vi "AddCommandFrame.vi"(5 "Command":T1 {"Data/Address/ByteCount" format="%.0x"}, 7 "Slave Address":u8 max=15 format="%.0x", 8 "error in (no error)":errorcluster, 9 "Number of Samples In":i32, 10 "Data Array In":u8[][](array[numeric]), 11 "RFFE_Data":T2 {"Toggle (high to low)" items=["0", "1", "Z", "L", "H", "X", "T", "V"]; "X Array" items=["0", "1", "Z", "L", "H", "X", "T", "V"]; "Z Array" items=["0", "1", "Z", "L", "H", "X", "T", "V"]; "L Array" items=["0", "1", "Z", "L", "H", "X", "T", "V"]; "H Array" items=["0", "1", "Z", "L", "H", "X", "T", "V"]; "One Array" items=["0", "1", "Z", "L", "H", "X", "T", "V"]; "Zero Array" items=["0", "1", "Z", "L", "H", "X", "T", "V"]}) -> (0 "error out":errorcluster, 1 "Number of Samples Out":i32, 2 "Data Array Out":u8[][](array[numeric]), 3 "Configuratation Out":T2 {"Toggle (high to low)" items=["0", "1", "Z", "L", "H", "X", "T", "V"]; "X Array" items=["0", "1", "Z", "L", "H", "X", "T", "V"]; "Z Array" items=["0", "1", "Z", "L", "H", "X", "T", "V"]; "L Array" items=["0", "1", "Z", "L", "H", "X", "T", "V"]; "H Array" items=["0", "1", "Z", "L", "H", "X", "T", "V"]; "One Array" items=["0", "1", "Z", "L", "H", "X", "T", "V"]; "Zero Array" items=["0", "1", "Z", "L", "H", "X", "T", "V"]})   [LabVIEW 2013]
doc: "Builds a MIPI RFFE command frame."
uses:
  Ctrls/RFFE_Data.ctl
  Ctrls/ClockDataChannels.ctl
  Ctrls/Commands.ctl
  Ctrls/Read_Write_Data.ctl
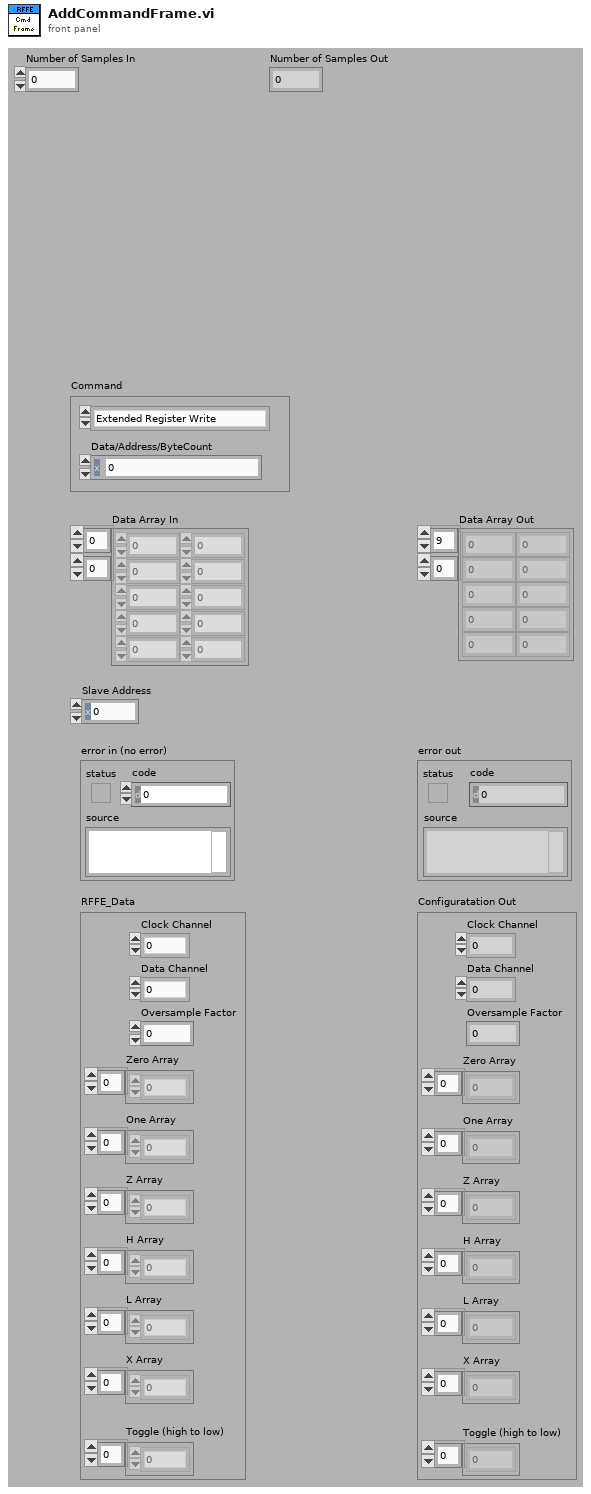
[diagram p1: front panel]
types:
  T1 = typedef "Commands.ctl" = cluster{"Command":enum16{"Extended Register Write", "Extended Register Read", "Extended Register Write Long", "Extended Register Read Long", "Register Write", "Register Read", "Register 0 Write"}, "Data/Address/ByteCount":u8}
  T2 = typedef "RFFE_Data.ctl" = cluster{"Clock Channel":T3, "Data Channel":T3, "Oversample Factor":u8, "Zero Array":u8[], "One Array":u8[], "Z Array ":u8[], "H Array":u8[], "L Array":u8[], "X Array":u8[], "Toggle (high to low)":u8[]}
  T3 = typedef "ClockDataChannels.ctl" = enum16{"0", "1"}
  T4 = enum16{"Extended Register Write", "Extended Register Read", "Extended Register Write Long", "Extended Register Read Long", "Register Write", "Register Read", "Register 0 Write"}
  T5 = typedef "Read_Write_Data.ctl" = cluster{"Data":u8, "Read/Write":enum16{"Read", "Write"}}
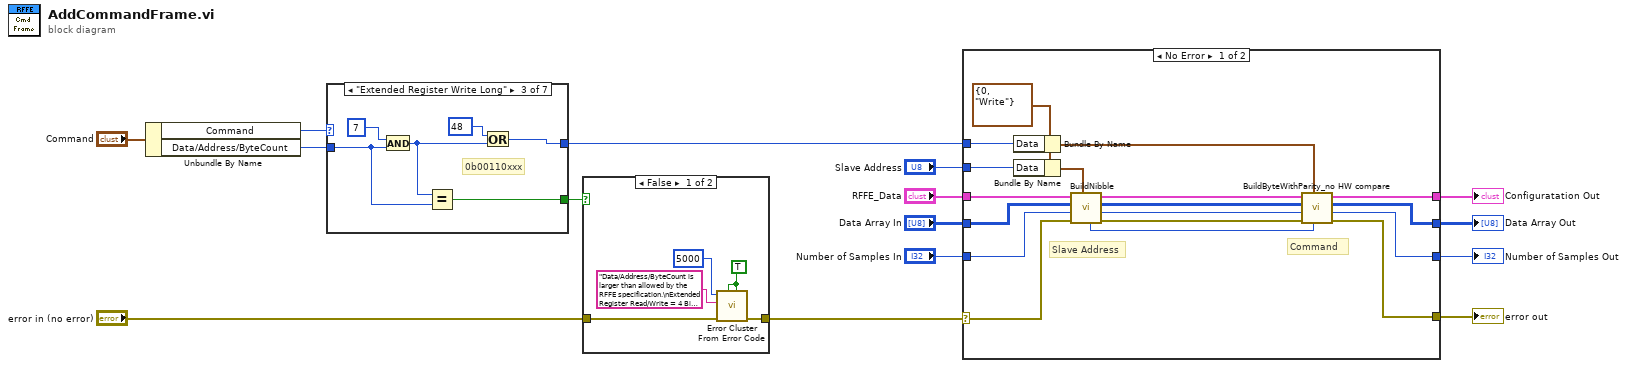
[diagram p0: block diagram]
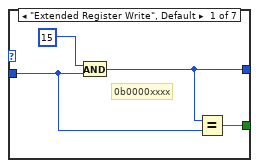
[diagram p3: hidden frame]
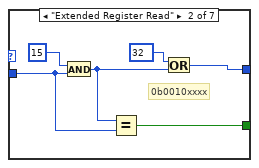
[diagram p4: hidden frame]
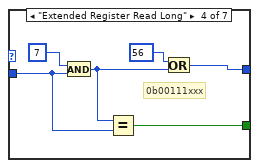
[diagram p5: hidden frame]
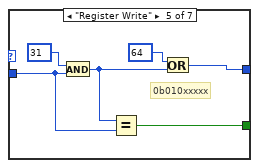
[diagram p6: hidden frame]
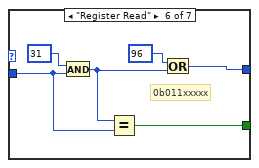
[diagram p7: hidden frame]
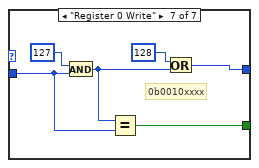
[diagram p8: hidden frame]
diagram:
  n1 = Unbundle By Name("Command") -> ("Command"=w9:T4, "Data/Address/ByteCount"=w8:u8)
  n2 = case shown="\"Extended Register Write Long\"" w9 {
    tunnel: w8 -> [w16 w20 w26 w32 w39 w45 w51]
    tunnel: [w17 w24 w29 w35 w41 w47 w53] -> w1
    tunnel: [w18 w22 w28 w34 w40 w44 w50] -> w7
    frame "Extended Register Write", Default {
      # "0b0000xxxx"
      n3 = And(x=u8 15, y=w16) -> (x .and. y?=w17:u8)
      n4 = Equal?(x=w17, y=w16) -> (x = y?=w18:bool)
    }
    frame "Extended Register Read" {
      # "0b0010xxxx"
      n5 = And(x=u8 15, y=w20) -> (x .and. y?=w21:u8)
      n6 = Equal?(x=w21, y=w20) -> (x = y?=w22:bool)
      n7 = Or(x=u8 32, y=w21) -> (x .or. y?=w24:u8)
    }
    frame "Extended Register Write Long" {
      # "0b00110xxx"
      n8 = And(x=u8 7, y=w26) -> (x .and. y?=w27:u8)
      n9 = Equal?(x=w27, y=w26) -> (x = y?=w28:bool)
      n10 = Or(x=u8 48, y=w27) -> (x .or. y?=w29:u8)
    }
    frame "Extended Register Read Long" {
      # "0b00111xxx"
      n11 = And(x=u8 7, y=w32) -> (x .and. y?=w33:u8)
      n12 = Equal?(x=w33, y=w32) -> (x = y?=w34:bool)
      n13 = Or(x=u8 56, y=w33) -> (x .or. y?=w35:u8)
    }
    frame "Register Write" {
      # "0b010xxxxx"
      n14 = And(x=u8 31, y=w39) -> (x .and. y?=w38:u8)
      n15 = Equal?(x=w38, y=w39) -> (x = y?=w40:bool)
      n16 = Or(x=u8 64, y=w38) -> (x .or. y?=w41:u8)
    }
    frame "Register Read" {
      # "0b011xxxxx"
      n17 = And(x=u8 31, y=w45) -> (x .and. y?=w46:u8)
      n18 = Equal?(x=w46, y=w45) -> (x = y?=w44:bool)
      n19 = Or(x=u8 96, y=w46) -> (x .or. y?=w47:u8)
    }
    frame "Register 0 Write" {
      # "0b0010xxxx"
      n20 = And(x=u8 127, y=w51) -> (x .and. y?=w52:u8)
      n21 = Equal?(x=w52, y=w51) -> (x = y?=w50:bool)
      n22 = Or(x=u8 128, y=w52) -> (x .or. y?=w53:u8)
    }
  }
  n23 = case shown="False" w7 {
    tunnel: [w59 w61] -> w5
    tunnel: "error in (no error)" -> [w60 w61]
    frame False {
      w56 = TRUE ("show call chain? (False)")
      n24 = call <vilib>:"Error Cluster From Error Code.vi"("is warning? (False)"=w56, "show call chain? (False)"=w56, "error in (no error)"=w60, "error message (\"\")"="Data/Address/ByteCount is larger than allowed by the RFFE specification.\nExtended Register Read/Write = 4 Bits\nExtended Register Read/Write Long = 3 Bits\nRegister Read/Write = 5 Bits\nRegister 0 Write = 7 Bits" ("error message (\"\")"), "error code (0)"=5000) -> ("error out"=w59:errorcluster)  [unwired: 4 in]
    }
    frame True {
    }
  }
  n25 = case shown="No Error" w5 {
    selector: w5 -> [w69 w83]
    tunnel: [w70 w83] -> w4
    tunnel: [w74 w82] -> w15
    tunnel: "RFFE_Data" -> [w75 w82]
    tunnel: [w72 w81] -> w3
    tunnel: "Data Array In" -> [w73 w81]
    tunnel: "Number of Samples In" -> [w68 w80]
    tunnel: [w71 w80] -> w2
    tunnel: "Slave Address" -> [w65 _]
    tunnel: w1 -> [w66 _]
    frame No Error {
      w64 = T5 {"Data"=0, "Read/Write"=enum."Write"} ("Read/Write Data")
      # "Command"
      # "Slave Address"
      n26 = Bundle By Name(cluster=w64, "Data"=w66) -> (w62:T5)
      n27 = Bundle By Name(cluster=w64, "Data"=w65) -> (w63:T5)
      n28 = call "BuildNibble.vi"("Read/Write Data"=w63, "error in (no error)"=w69, "Number of Samples In"=w68, "Data Array In"=w73, "RFFE_Data In"=w75) -> ("error out"=w79:errorcluster, "Number of Samples Out"=w78:i32, "Data Array Out"=w77:u8[][], "RFFE_Data Out"=w76:T2, "Parity Out"=w67:u8)  [unwired: 2 in]
      n29 = call "BuildByteWithParity_no HW compare.vi"("Parity Count In"=w67, "Read/Write Data"=w62, "error in"=w79, "Number of Samples In"=w78, "Data Array In"=w77, "RFFE_Data In"=w76) -> ("error out"=w70:errorcluster, "Number of Samples Out"=w71:i32, "Data Array Out"=w72:u8[][], "RFFE_Data Out"=w74:T2)  [unwired: 1 in, 1 out]
    }
    frame Error {
    }
  }
  "error out" <- w4
  "Configuratation Out" <- w15
  "Data Array Out" <- w3
  "Number of Samples Out" <- w2
